vi "TempsBalayageGen.vi"(0 "NbPoints":i32, 1 "NbCourbes":i32=1 caption="Nombre de Balayages" min=0 max=20 step=1, 3 "error in (no error)":errorcluster, 4 "Dwell":u32=1000 caption="Dwell (ms)" min=1 max=100000 step=1) -> (5 "Temps(s)":dbl, 6 "error out":errorcluster)   [LabVIEW 2019]
doc: "Ce Vi sert à calculer le temps estimé de balayage, en fonctions des paramètres choisis."
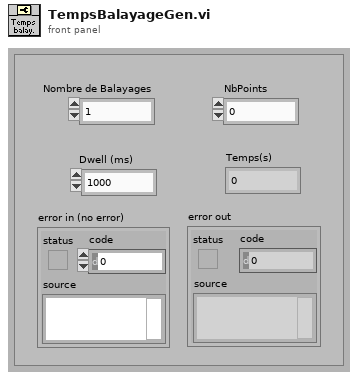
[diagram p1: front panel]
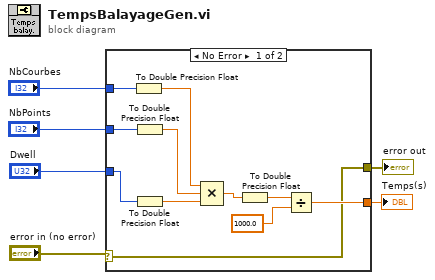
[diagram p0: block diagram]
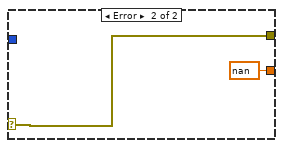
[diagram p2: hidden frame]
diagram:
  n1 = case shown="No Error" "error in (no error)" {
    selector: "error in (no error)" -> [w9 w19]
    tunnel: "NbPoints" -> [w17 _]
    tunnel: "NbCourbes" -> [w16 _]
    tunnel: "Dwell" -> [w8 _]
    tunnel: [w11 nan] -> w3
    tunnel: [w9 w19] -> w1
    frame No Error {
      n2 = To Double Precision Float(number=w16) -> (double precision float=w14:dbl)
      n3 = To Double Precision Float(number=w17) -> (double precision float=w15:dbl)
      n4 = To Double Precision Float(number=w8) -> (double precision float=w7:dbl)
      n5 = Compound Arithmetic op=MULTIPLY(w14, w15, w7) -> (w13:dbl)
      n6 = To Double Precision Float(number=w13) -> (double precision float=w10:dbl)
      n7 = Divide(x=w10, y=1000.0) -> (x/y=w11:dbl)
    }
    frame Error {
    }
  }
  "Temps(s)" <- w3
  "error out" <- w1
